vi "CPC3752.vi"() -> ()   [LabVIEW 2017]
uses:
  <vilib>/regexp/Match Regular Expression.xnode
panel:
  out "value 2":T1
  out "whole match":string
  in  "stop":bool
  out "data out 4":string
  out "data out 3":string
  out "value":T2
  out "data out":string
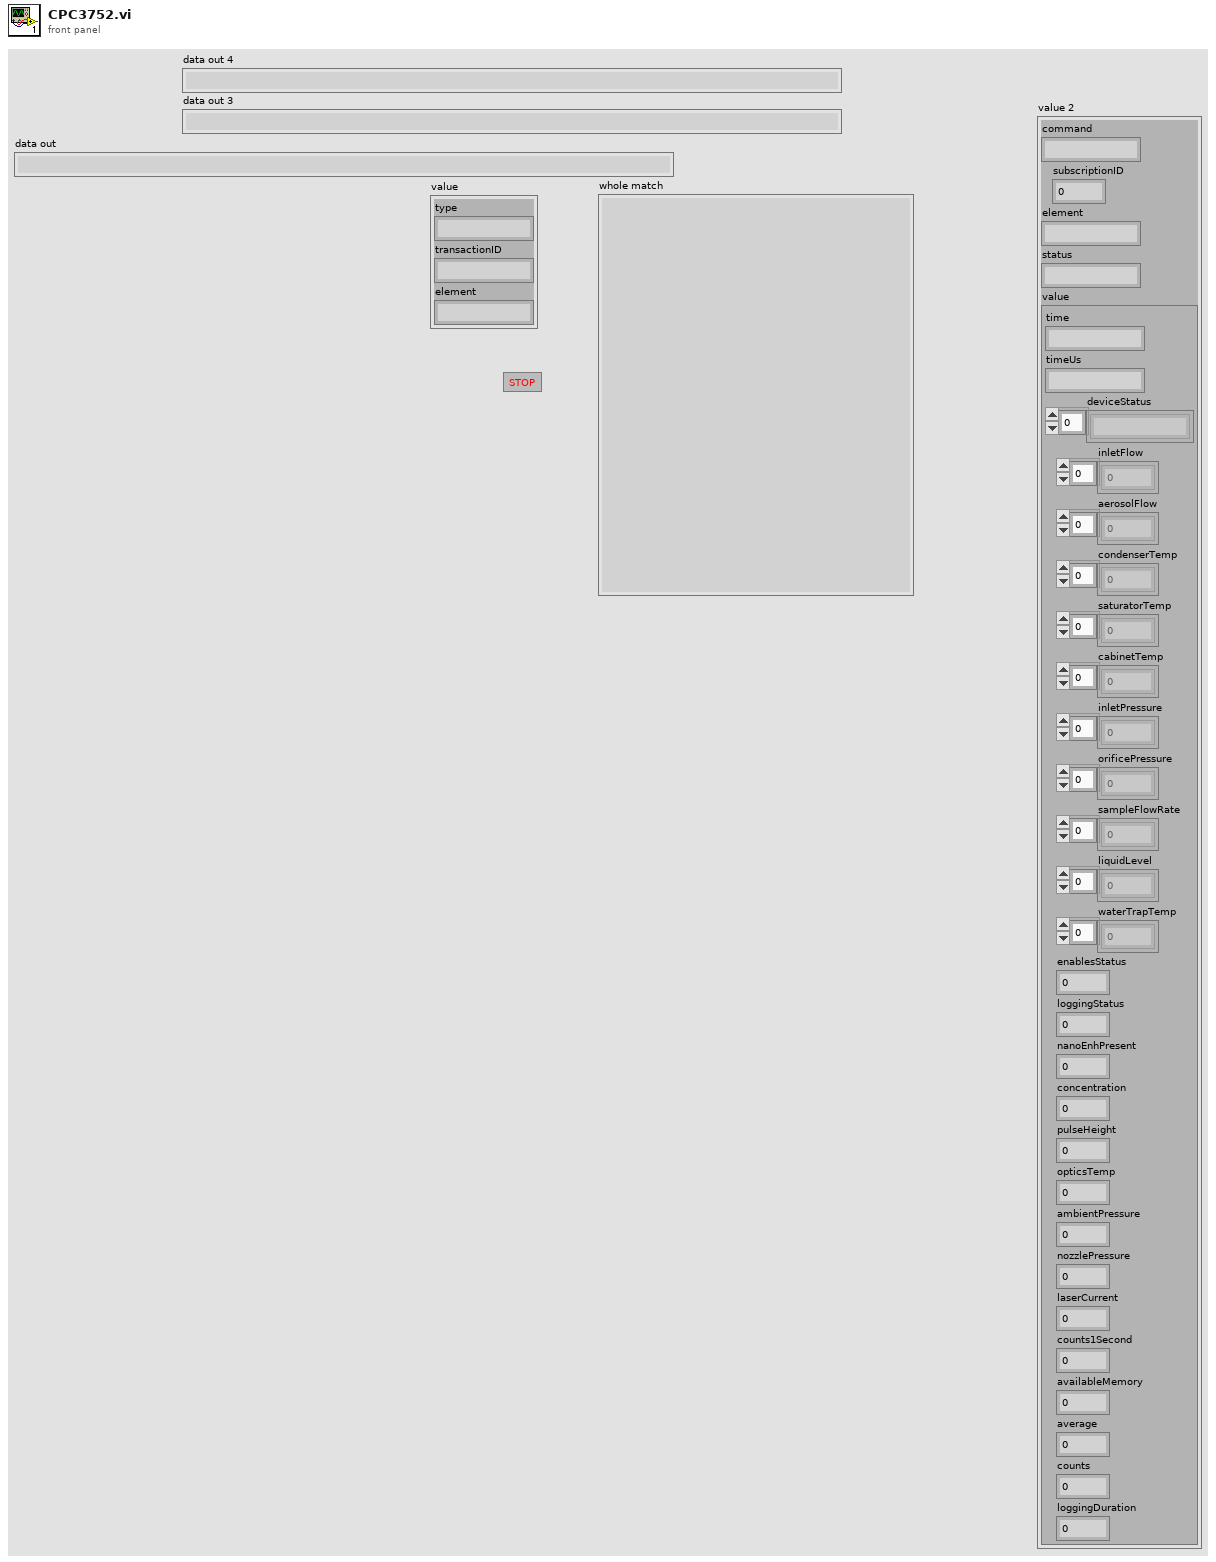
[diagram p1: front panel]
types:
  T1 = cluster{"command":string, "subscriptionID":i32, "element":string, "status":string, "value":cluster{"time":string, "timeUs":string, "deviceStatus":string[], "inletFlow":dbl[], "aerosolFlow":dbl[], "condenserTemp":dbl[], "saturatorTemp":dbl[], "cabinetTemp":dbl[], "inletPressure":dbl[], "orificePressure":dbl[], "sampleFlowRate":dbl[], "liquidLevel":dbl[], "waterTrapTemp":dbl[], "enablesStatus":i32, "loggingStatus":i32, "nanoEnhPresent":i32, "concentration":dbl, "pulseHeight":i32, "opticsTemp":dbl, "ambientPressure":dbl, "nozzlePressure":dbl, "laserCurrent":dbl, "counts1Second":dbl, "availableMemory":dbl, "average":dbl, "counts":dbl, "loggingDuration":dbl}}
  T2 = cluster{"type":string, "transactionID":string, "element":string}
  T3 = enum16{"Standard", "Buffered", "CRLF", "Immediate"}
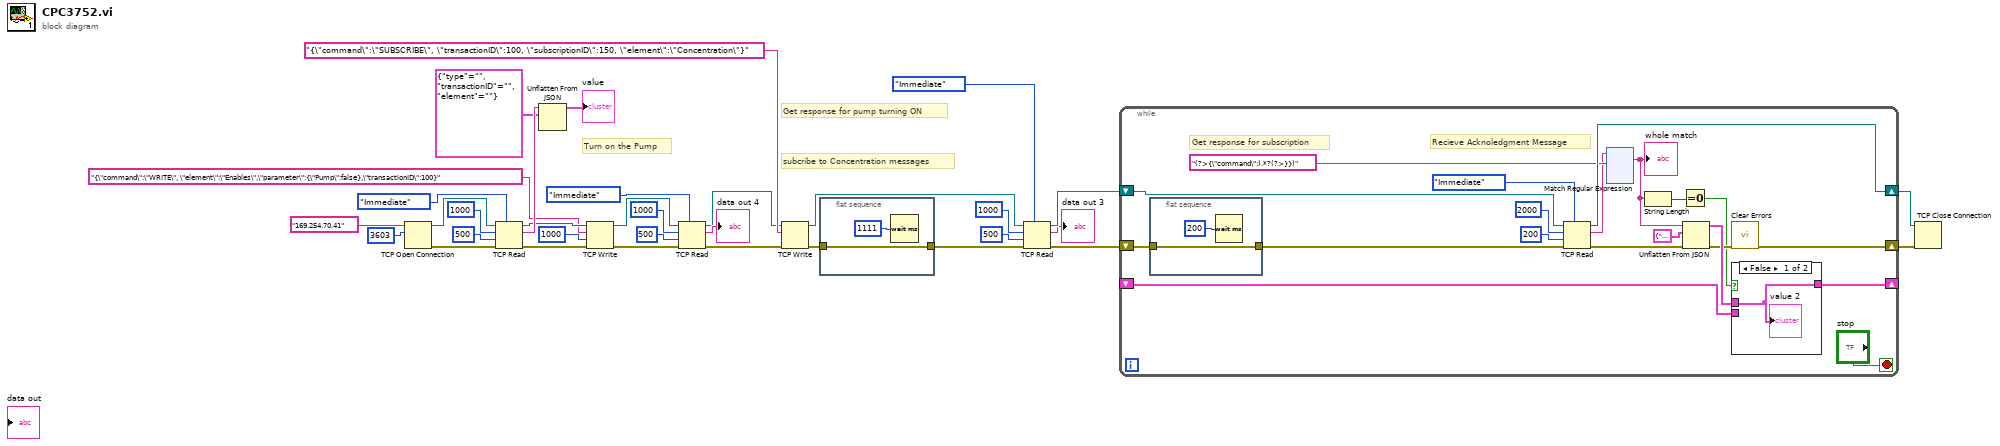
[diagram p0: block diagram]
diagram:
  # "Get response for pump turning ON"
  # "subcribe to Concentration messages"
  # "Turn on the Pump"
  n1 = TCP Open Connection(address="169.254.70.41", remote port or service name=u16 3603) -> (connection ID=w31:refnum<k5>, error out=w32:errorcluster)  [unwired: 3 in]
  n2 = TCP Read(connection ID=w31, bytes to read=1000, error in (no error)=w32, 7:T3."Immediate" ("mode (standard)"), 9:500 ("timeout ms (25000)")) -> (connection ID out=w24:refnum<k5>, data out=w27:string, error out=w23:errorcluster)
  n3 = Unflatten From JSON(JSON string=w27, type and defaults=T2 {"type"="", "transactionID"="", "element"=""}) -> (value=→"value":T2)  [unwired: 5 in, 1 out]
  n4 = TCP Write(connection ID=w24, data in="{\"command\":\"WRITE\", \"element\":\"Enables\",\"parameter\":{\"Pump\":false},\"transactionID\":100}", error in (no error)=w23, 9:1000 ("timeout ms (25000)")) -> (connection ID out=w4:refnum<k5>, error out=w6:errorcluster)  [unwired: 1 out]
  n5 = TCP Read(connection ID=w4, bytes to read=1000, error in (no error)=w6, 7:T3."Immediate" ("mode (standard)"), 9:500 ("timeout ms (25000)")) -> (connection ID out=w3:refnum<k5>, data out=→"data out 4":string, error out=w5:errorcluster)
  n6 = TCP Write(connection ID=w3, data in="{\"command\":\"SUBSCRIBE\", \"transactionID\":100, \"subscriptionID\":150, \"element\":\"Concentration\"}", error in (no error)=w5) -> (connection ID out=w19:refnum<k5>, error out=w11:errorcluster)  [unwired: 1 in, 1 out]
  n7 = flat-sequence {
    tunnel: w11 -> [w35]
    tunnel: [w35] -> w10
    frame #0 {
      n8 = Wait (ms)(milliseconds to wait=u32 1111) -> ()  [unwired: 1 out]
    }
  }
  n9 = TCP Read(connection ID=w19, bytes to read=1000, error in (no error)=w10, 7:T3."Immediate" ("mode (standard)"), 9:500 ("timeout ms (25000)")) -> (connection ID out=w14:refnum<k5>, data out=→"data out 3":string, error out=w12:errorcluster)
  n10 = while {
    shift-right: [w52] -> w13
    shift-left: w14 -> [w56]
    shift-right: [w42] -> w15
    shift-left: w12 -> [w51]
    shift-right: [w38] -> _
    shift-left: _ -> [w37]
    stop <- "stop" stop-if-true
    # "Get response for subscription"
    # "Recieve Acknoledgment Message"
    n11 = flat-sequence {
      tunnel: w51 -> [w173]
      tunnel: [w173] -> w50
      frame #0 {
        n12 = Wait (ms)(milliseconds to wait=u32 200) -> ()  [unwired: 1 out]
      }
    }
    n13 = TCP Read(connection ID=w56, bytes to read=2000, error in (no error)=w50, 7:T3."Immediate" ("mode (standard)"), 9:200 ("timeout ms (25000)")) -> (connection ID out=w52:refnum<k5>, data out=w47:string, error out=w43:errorcluster)
    n14 = xnode "Match Regular Expression"("input string"=w47, "regular expression"="(?>{\"command\":).*?(?>}})") -> ("whole match"=w41:string)  [unwired: 4 in, 4 out]
    "whole match" <- w41
    n15 = String Length(string=w41) -> (length=w40:i32)
    n16 = Equal To 0?(x=w40) -> (x = 0?=w39:bool)
    n17 = Unflatten From JSON(JSON string=w41, type and defaults=T1 {"command"="", "subscriptionID"=0, "element"="", "status"="", "value"={"time"="", "timeUs"="", "deviceStatus"=[], "inletFlow"=[], "aerosolFlow"=[], "condenserTemp"=[], "saturatorTemp"=[], "cabinetTemp"=[], "inletPressure"=[], "orificePressure"=[], "sampleFlowRate"=[], "liquidLevel"=[], "waterTrapTemp"=[], "enablesStatus"=0, "loggingStatus"=0, "nanoEnhPresent"=0, "concentration"=0.0, "pulseHeight"=0, "opticsTemp"=0.0, "ambientPressure"=0.0, "nozzlePressure"=0.0, "laserCurrent"=0.0, "counts1Second"=0.0, "availableMemory"=0.0, "average"=0.0, "counts"=0.0, "loggingDuration"=0.0}}, error in (no error)=w43) -> (value=w45:T1, error out=w44:errorcluster)  [unwired: 4 in]
    n18 = call <vilib>:"Clear Errors.vi"("error in (no error)"=w44) -> ("error out"=w42:errorcluster)  [unwired: 5 in, 1 out]
    n19 = case shown="False" w39 {
      tunnel: w45 -> [w57 _]
      tunnel: [w57 w58] -> w38
      tunnel: w37 -> [_ w58]
      frame False {
        "value 2" <- w57
      }
      frame True {
      }
    }
  }
  n20 = TCP Close Connection(connection ID=w13, error in (no error)=w15) -> ()  [unwired: 1 in, 2 out]
